vi "get and check open config.vi"(9 "App Name":string, 11 "Working Directory In":path) -> (0 "error out":errorcluster, 1 "ConnectionType":string="LJM_ctANY", 2 "DeviceType":string="LJM_dtANY", 3 "Working Directory Out":path, 4 "Identifier":string="LJM_idANY", 6 "Device Open Config File Name":string, 8 "New Open Config?":bool=TRUE)   [LabVIEW 2025]
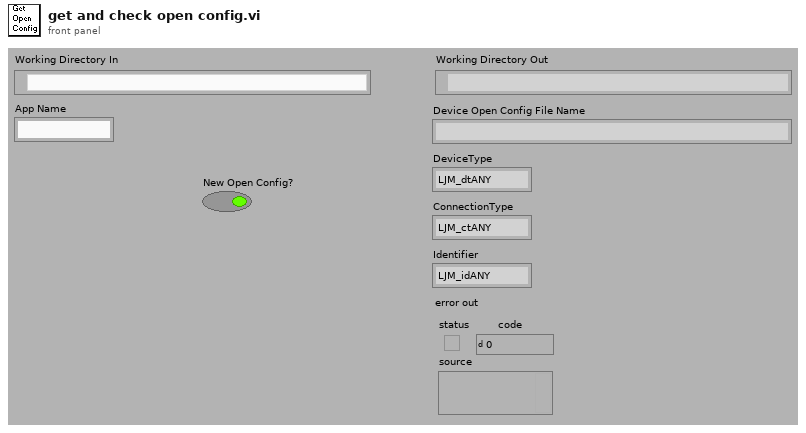
[diagram p1: front panel]
types:
  T1 = enum16{"Left Button", "Center Button", "Right Button", "Window Close"}
  T2 = enum32{"existing file", "new file", "new or existing file", "existing dir", "new dir", "new or existing dir", "existing file (use LLBs)", "new file (use LLBs)", "new or existing file (use LLBs)", "new or existing file or directory (use LLBs)"}
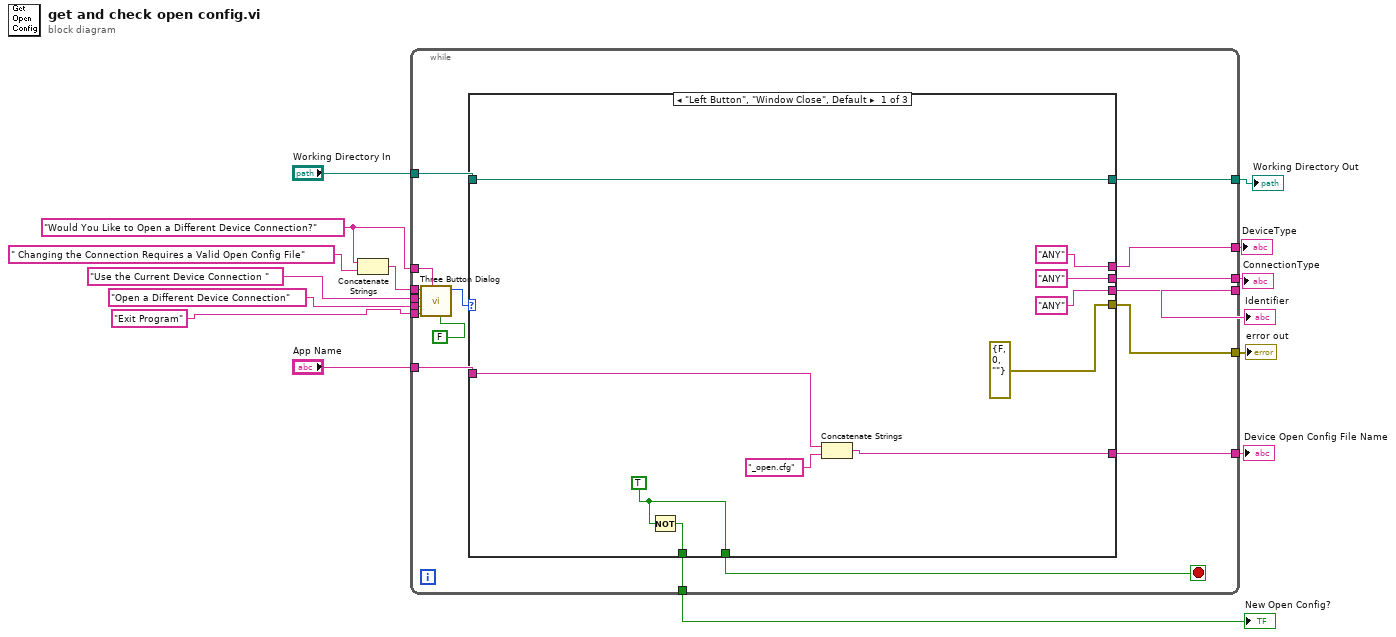
[diagram p0: block diagram]
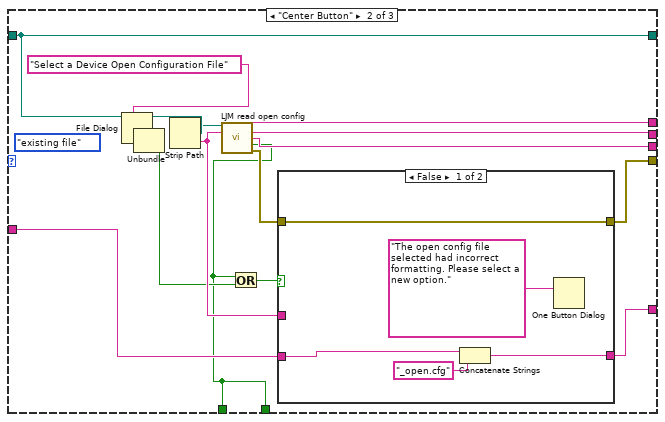
[diagram p2: hidden frame]
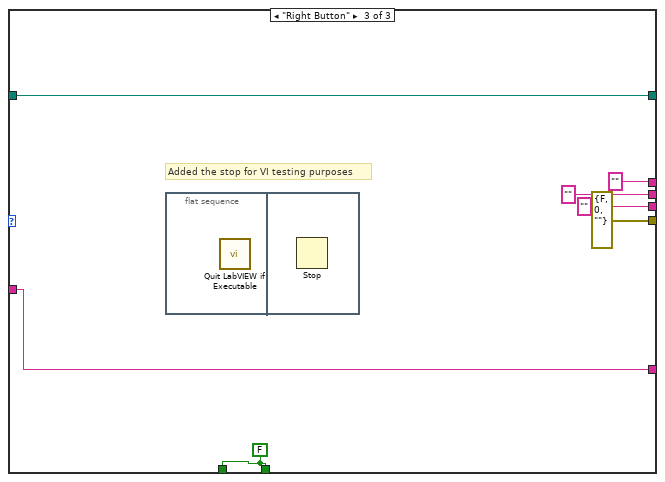
[diagram p4: hidden frame]
diagram:
  w4 = "Would You Like to Open a Different Device Connection?" ("message")
  n1 = Concatenate Strings(w4, " Changing the Connection Requires a Valid Open Config File" ("message")) -> (w2:string)
  n2 = while {
    tunnel: "Working Directory In" -> [w32]
    tunnel: [w31] -> w14
    tunnel: "App Name" -> [w30]
    tunnel: [w29] -> w12
    tunnel: [w28] -> w11
    tunnel: [w27] -> w10
    tunnel: [w26] -> w9
    tunnel: [w25] -> w8
    tunnel: w4 -> [w18]
    tunnel: "Use the Current Device Connection " ("F button name (\"Cancel\")") -> [w22]
    tunnel: "Open a Different Device Connection" ("T button name (\"OK\")") -> [w21]
    tunnel: "Exit Program" ("Right Button Text (\"Cancel\")") -> [w20]
    tunnel: w2 -> [w17]
    tunnel: [w16] -> w1
    stop <- w24 stop-if-true
    n3 = call <vilib>:"Three Button Dialog.vi"("Allow user to close window? (TRUE)"=FALSE, "Window Title (\"\")"=w18, "Right Button Text (\"Cancel\")"=w20, "Center Button Text (\"No\")"=w21, "Left Button Text (\"Yes\")"=w22, "message"=w17) -> ("Which Button?"=w23:T1)  [unwired: 5 in]
    n4 = case shown="\"Left Button\", \"Window Close\", Default" w23 {
      tunnel: w32 -> [w39 w49 w67]
      tunnel: [w40 w53 w72] -> w31
      tunnel: w30 -> [w41 w54 w72]
      tunnel: [errorcluster {"status"=FALSE, "code"=0, "source"=""} ("error out") w50 errorcluster {"status"=FALSE, "code"=0, "source"=""} ("error out")] -> w29
      tunnel: ["ANY" ("DeviceType") w57 "" ("Identifier")] -> w28
      tunnel: ["ANY" ("DeviceType") w56 "" ("ConnectionType")] -> w27
      tunnel: ["ANY" ("DeviceType") w55 "" ("DeviceType")] -> w26
      tunnel: [w39 w49 w67] -> w25
      tunnel: [w34 w44 w66] -> w24
      tunnel: [w33 w44 w66] -> w16
      frame "Left Button", "Window Close", Default {
        w34 = TRUE ("Good Open Config")
        n5 = Not(x=w34) -> (.not. x?=w33:bool)
        n6 = Concatenate Strings(w41, "_open.cfg" ("filename")) -> (w40:string)
      }
      frame "Center Button" {
        (unwired) T2."existing file" ("select mode (2)")
        n7 = File Dialog(7:"Select a Device Open Configuration File" ("Substring"), 11:w49) -> (0:w43:errorcluster, 1:w45:bool, 3:w52:path)  [unwired: 5 in, 1 out]
        n8 = Unbundle(w43) -> ()  [unwired: 3 out]
        n9 = Strip Path(path=w52) -> (stripped path=w48:path, name=w47:string)
        n10 = call "LJM read open config.vi"("Working Directory"=w48, "filename"=w47) -> ("DeviceType"=w55:string, "ConnectionType"=w56:string, "Identifier"=w57:string, "Good Open Config"=w44:bool, "error out"=w51:errorcluster)  [unwired: 9 in]
        n11 = Or(x=w44, y=w45) -> (x .or. y?=w46:bool)
        n12 = case shown="False" w46 {
          tunnel: w54 -> [w61 _]
          tunnel: [w60 w65] -> w53
          tunnel: w47 -> [_ w65]
          tunnel: w51 -> [w59 w64]
          tunnel: [w59 w64] -> w50
          frame False {
            n13 = Concatenate Strings(w61, "_open.cfg" ("string")) -> (w60:string)
            n14 = One Button Dialog(message="The open config file selected had incorrect formatting. Please select a new option.") -> ()  [unwired: 1 in, 1 out]
          }
          frame True {
          }
        }
      }
      frame "Right Button" {
        w66 = FALSE ("Good Open Config")
        # "Added the stop for VI testing purposes"
        n15 = flat-sequence {
          frame #0 {
            n16 = call "Quit LabVIEW if Executable.vi"() -> ()  [unwired: 1 in]
          }
          frame #1 {
            n17 = Stop() -> ()  [unwired: 1 in]
          }
        }
      }
    }
  }
  "Device Open Config File Name" <- w14
  "DeviceType" <- w9
  "ConnectionType" <- w10
  "Identifier" <- w11
  "error out" <- w12
  "Working Directory Out" <- w8
  "New Open Config?" <- w1
